vi "Get CLST Configuration.vi"(2 "gen":refnum<class "niUSRP Tx DSP v2 FPGA.lvclass">=refnum) -> (4 "list mode.clst.source type":T1, 6 "list mode.event.ready for CLST":bool, 8 "list mode.clst.sw trigger":bool, 10 "list mode.clst.rising edge":bool)   [LabVIEW 2023]
uses:
  <vilib>/rvi/DataTransferAndStorage/Container/XNode/niFpgaContainer.xnode
  <vilib>/rvi/DataTransferAndStorage/Register/Emulation/niFpgaRegisterEmulationRefIn.vi
  <instrlib>/niVST/List Mode/Interface/v1/FPGA/niVST List Mode Interface v1 FPGA.lvclass
  <instrlib>/niUSRP/Reference FPGA/Tx DSP/niUSRP Tx DSP v2 FPGA.lvclass
  <instrlib>/niVST/Reference FPGA/FPGA/Tx DSP/niUSRP Tx DSP v2 FPGA.lvclass
  <instrlib>/niVST/Reference FPGA/FPGA/Shared/v1/Public/Typedefs/Trigger Source Type.ctl
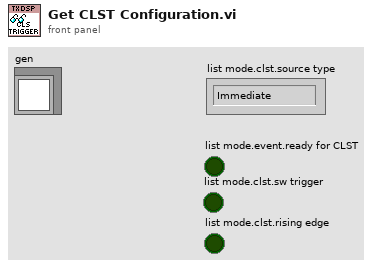
[diagram p1: front panel]
types:
  T1 = typedef "niVST Shared v1 FPGA.lvclass/Trigger Source Type.ctl" = enum8{"Immediate", "Software", "Digital Edge", "IQ Power Edge", "Digital Level", "IQ Analog Edge", "Custom"}
  T2 = typedef "niUSRP Tx DSP v2 FPGA.lvclass/Tx DSP Shared Registers.ctl" = cluster{"reset":refnum<k21>, "reset.done":refnum<k21>, "ignore overflows":refnum<k21>, "overflow":refnum<k21>, "overflow.clear":refnum<k21>, "pipeline delay":refnum<k21>, "group delay (output samples)":refnum<k21>, "blanking delay.data clock ticks":refnum<k21>, "dynamic delay.data clock ticks":refnum<k21>, "dynamic delay.samples":refnum<k21>, "bypass EQ":refnum<k21>, "inject idle into path":refnum<k21>, "TxDspEnabled":refnum<k21>}
  T3 = cluster{"source type":refnum<k21>, "rising edge":refnum<k21>, "sw trigger":refnum<k21>, "min import pulse width (clocks)":refnum<k21>, "min export pulse width (clocks)":refnum<k21>}
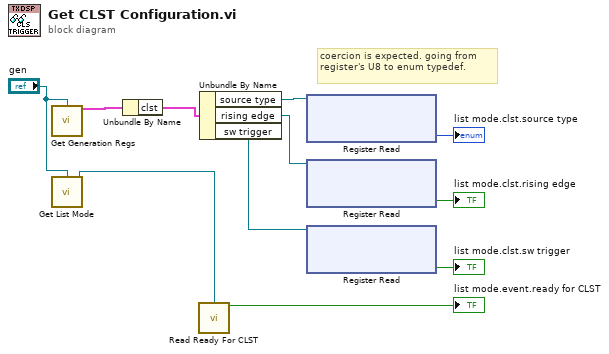
[diagram p0: block diagram]
diagram:
  # "coercion is expected. going from register's U8 to enum typedef."
  n1 = call-dynamic "Get Generation Regs.vi"("gen"="gen") -> ("dsp"=w11:T2)  [unwired: 14 in]
  n2 = call-dynamic "Get List Mode.vi"("gen"="gen") -> ("list mode"=w3:refnum<class "niVST List Mode Interface v1 FPGA.lvclass">)  [unwired: 14 in]
  n3 = Unbundle By Name(w11) -> ("clst"=w10:T3)
  n4 = call-dynamic "Read Ready For CLST.vi"("list mode"=w3) -> ("ready for CLST"=→"list mode.event.ready for CLST":bool)  [unwired: 14 in]
  n5 = Unbundle By Name(w10) -> ("source type"=w9:refnum<k21>, "rising edge"=w8:refnum<k21>, "sw trigger"=w2:refnum<k21>)
  n6 = xnode ("Register Read")("Register In"=w9) -> ("Data"=→"list mode.clst.source type":u8)  [unwired: 1 out]
  n7 = xnode ("Register Read")("Register In"=w8) -> ("Data"=→"list mode.clst.rising edge":bool)  [unwired: 1 out]
  n8 = xnode ("Register Read")("Register In"=w2) -> ("Data"=→"list mode.clst.sw trigger":bool)  [unwired: 1 out]
